vi "Close Power Meter and Clear Cache.vi"(11 "error in (no error)":errorcluster) -> (15 "error out":errorcluster)   [LabVIEW 2023, in "RFFixtureCharact.Instruments.lvlib" / "Power Meter Factory.lvclass"]
uses:
  Power Meter Factory.lvclass
  Power Meter Base/Power Meter Base.lvclass
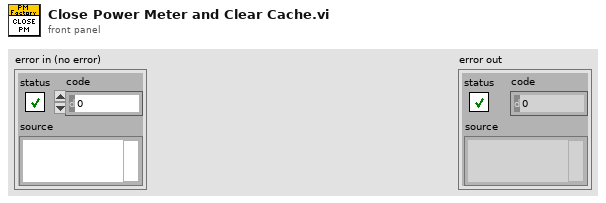
[diagram p1: front panel]
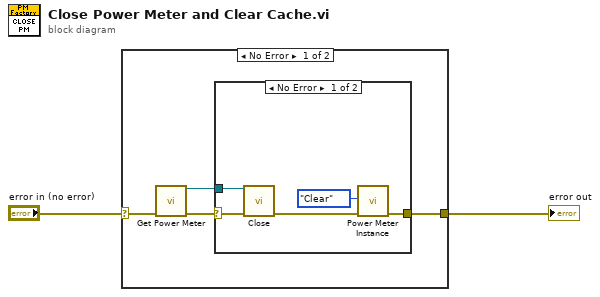
[diagram p0: block diagram]
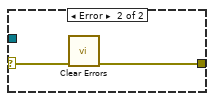
[diagram p2: hidden frame]
diagram:
  n1 = case shown="No Error" "error in (no error)" {
    selector: "error in (no error)" -> [w5 w14]
    tunnel: [w6 w14] -> w1
    frame No Error {
      n2 = call "Get Power Meter.vi"("error in (no error)"=w5) -> ("Power Meter Base out"=w3:refnum<class "Power Meter Base.lvclass">, "error out"=w4:errorcluster)  [unwired: 13 in]
      n3 = case shown="No Error" w4 {
        selector: w4 -> [w10 w13]
        tunnel: [w8 w12] -> w6
        tunnel: w3 -> [w9 _]
        frame No Error {
          n4 = call-dynamic "Close.vi"("Power Meter Base in"=w9, "error in (no error)"=w10) -> ("error out"=w11:errorcluster)  [unwired: 12 in, 1 out]
          n5 = call "Power Meter Instance.vi"("Operation"=enum16{"Read", "Write", "Clear"}."Clear", "error in (no error)"=w11) -> ("error out"=w8:errorcluster)  [unwired: 11 in, 2 out]
        }
        frame Error {
          n6 = call <vilib>:"Clear Errors.vi"("error in (no error)"=w13) -> ("error out"=w12:errorcluster)  [unwired: 5 in, 1 out]
        }
      }
    }
    frame Error {
    }
  }
  "error out" <- w1
